vi "IMAQ FPGA Camera Link Pixel Bus to Vision Pixel Bus U16x1.vi"(5 "Reset Overflow":bool, 6 "Ready for Output":bool=TRUE, 7 "Overflow In":bool, 8 "Input Valid":bool=TRUE, 9 "Frame Valid In":bool, 10 "Line Valid In":bool, 11 "Pixel In":u16) -> (0 "Output Valid":bool, 2 "Acquisition Overflow":bool, 3 "Vision Pixel Bus Out":T1)   [LabVIEW 2017]
doc: "The Pixel Bus to Vision Pixel Bus takes the <B>Pixel In</B> and the timing signals (Line Valid, Frame Valid, and Input Valid) and converts them to the data structure used by Vision FPGA functions where the Line Valid and Frame Valid are part of the <B>Vision Pixel Bus Out</B> data structure.\n\nIf Ready For Output is ever False (i.e. downstream VIs are not ready for new pixel data), and this VI is about to output a valid Vision Pixel Bus, the Acquisition Overflow will assert and stay high to indicate pixel data was lost. The CameraLink pixel bus can not be slowed down, so the downstream processing VIs and transfer VIs need to ensure they can handle the CameraLink throughput to avoid missing pixels.\n\nThis VI requires a cycle to add End of Line and another cycle to add End of Image at the end of every image. This means there needs to be at least two blanking cycles between frames.s"
uses:
  <vilib>/visionFPGA/Controls/IMAQ FPGA Pixel Bus u16x1.ctl
  <vilib>/visionFPGA/Basics/Camera Link Acquisition/Controls/IMAQ FPGA Camera Link Pixel Bus to Vision Bus State.ctl
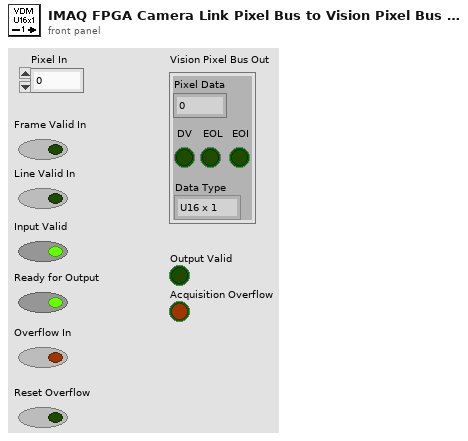
[diagram p1: front panel]
types:
  T1 = typedef "IMAQ FPGA Pixel Bus u16x1.ctl" = cluster{"Pixel Data":u16, "DV":bool, "EOL":bool, "EOI":bool, "Data Type":enum16{"U16 x 1"}}
  T2 = typedef "IMAQ FPGA Camera Link Pixel Bus to Vision Bus State.ctl" = enum16{"WaitForFirstPixel", "WaitForEndOfLine", "WaitForStartofNextLineOrEndOfImage", "HandleEndOfImage"}
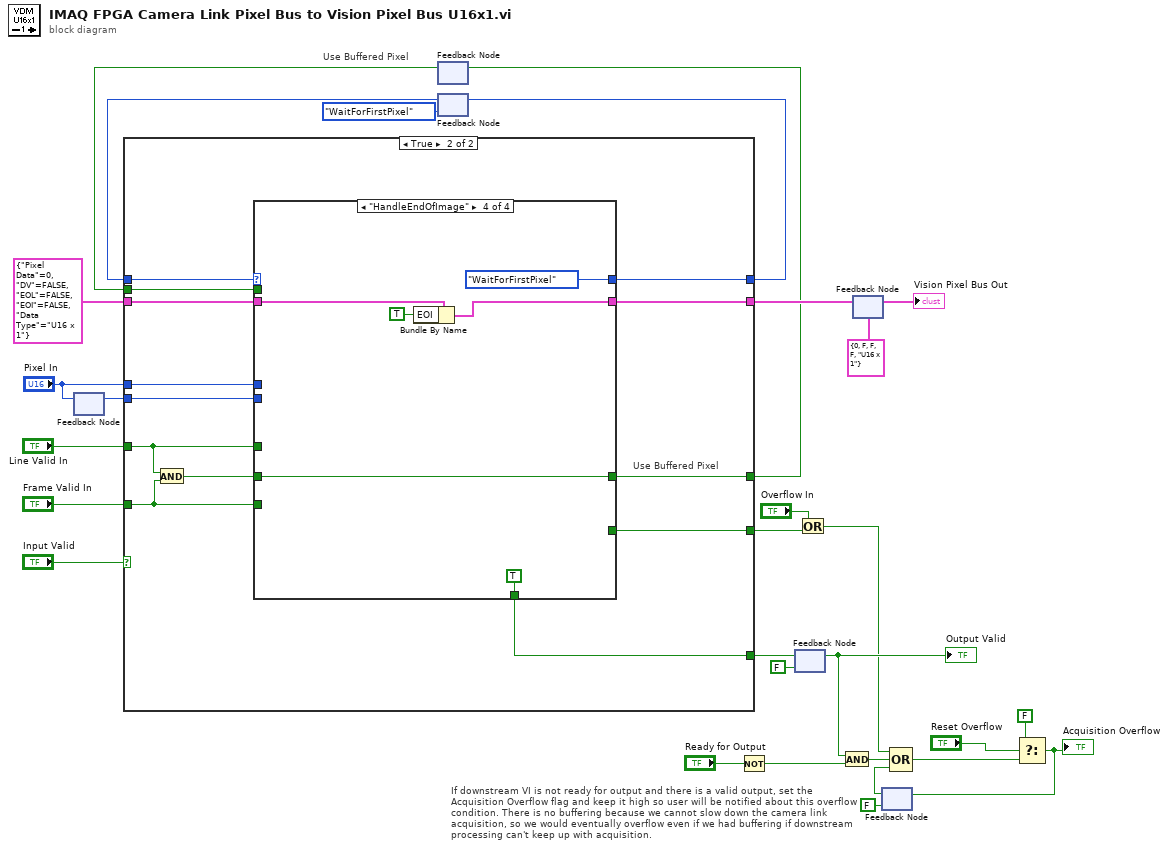
[diagram p0: block diagram]
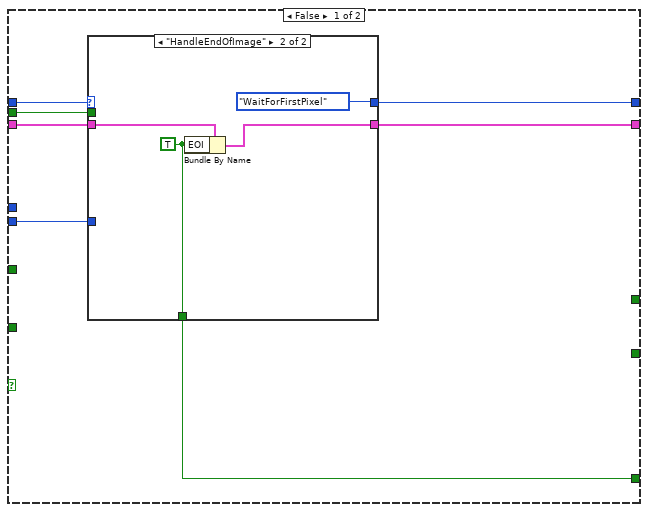
[diagram p2: hidden frame]
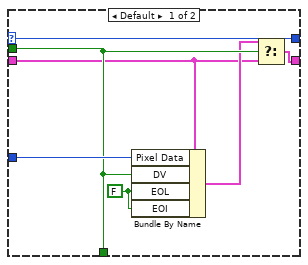
[diagram p3: hidden frame]
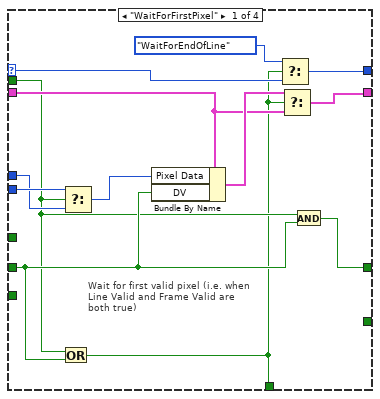
[diagram p4: hidden frame]
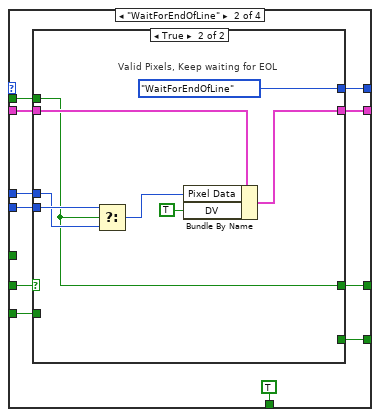
[diagram p5: hidden frame]
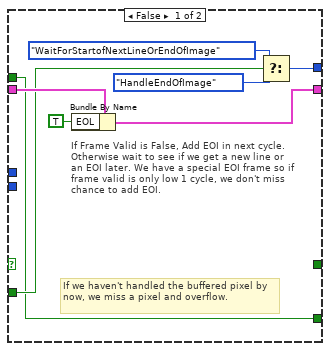
[diagram p6: hidden frame]
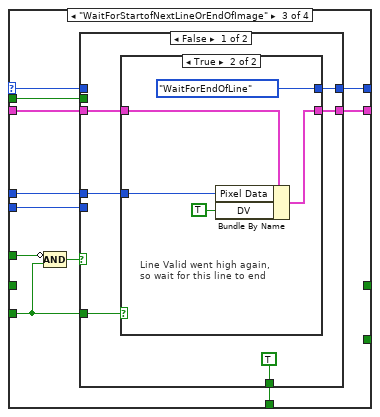
[diagram p7: hidden frame]
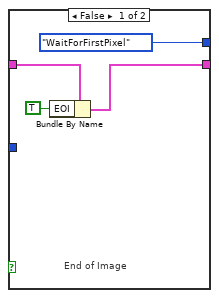
[diagram p8: hidden frame]
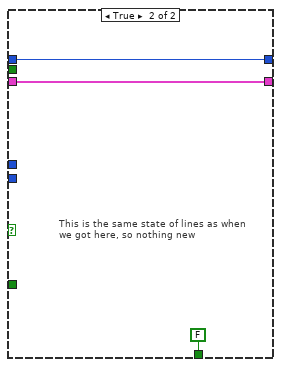
[diagram p9: hidden frame]
diagram:
  # "Use Buffered Pixel"
  # "If downstream VI is not ready for output and there is a valid output, set the Acquisition Overflow flag and keep it high so user will be notified about this overflow condition. There is no buffering because we cannot slow down the camera link acquisition, so we would eventually overflow even if we had buffering if downstream processing can't keep up with acquisition."
  n1 = feedback #1() -> (w7:u16)  [unwired: 1 in]
  n2 = feedback-in #1("Pixel In") -> ()
  n3 = feedback #2() -> (w8:bool)  [unwired: 1 in]
  n4 = feedback #3(IMAQ_FPGA_Camera_Link_Pixel_Bus_to_Vision_Bus_State."WaitForFirstPixel") -> (w11:T2)
  n5 = case shown="True" "Input Valid" {
    tunnel: [w32 w54] -> w25
    tunnel: "Line Valid In" -> [_ w56]
    tunnel: "Frame Valid In" -> [_ w55]
    tunnel: [w34 w59] -> w24
    tunnel: T1 {"Pixel Data"=0, "DV"=FALSE, "EOL"=FALSE, "EOI"=FALSE, "Data Type"=enum."U16 x 1"} ("Vision Pixel Bus Out") -> [w35 w60]
    tunnel: "Pixel In" -> [_ w58]
    tunnel: [w33 w53] -> w12
    tunnel: w11 -> [w36 w52]
    tunnel: [_ w51] -> w10
    tunnel: w8 -> [w31 w50]
    tunnel: w7 -> [w30 w49]
    tunnel: [_ w48] -> w5
    frame False {
      n6 = case shown="\"HandleEndOfImage\"" w36 {
        selector: w36 -> [w43 _]
        tunnel: w35 -> [w38 w47]
        tunnel: [w37 w46] -> w34
        tunnel: [w43 IMAQ_FPGA_Camera_Link_Pixel_Bus_to_Vision_Bus_State."WaitForFirstPixel"] -> w33
        tunnel: [w40 w44] -> w32
        tunnel: w31 -> [w40 _]
        tunnel: w30 -> [w42 _]
        frame Default {
          w41 = FALSE ("EOL")
          n7 = Bundle By Name(cluster=w38, "Pixel Data"=w42, "DV"=w40, "EOL"=w41, "EOI"=w41) -> (w39:T1)
          n8 = Select(t=w39, s=w40, f=w38) -> (s? t:f=w37:T1)
        }
        frame "HandleEndOfImage" {
          w44 = TRUE ("EOI")
          n9 = Bundle By Name(cluster=w47, "EOI"=w44) -> (w46:T1)
        }
      }
    }
    frame True {
      # "Use Buffered Pixel"
      n10 = And(x=w56, y=w55) -> (x .and. y?=w57:bool)
      n11 = case shown="\"HandleEndOfImage\"" w52 {
        selector: w52 -> [w72 _ w109 _]
        tunnel: [w73 w80 w108 IMAQ_FPGA_Camera_Link_Pixel_Bus_to_Vision_Bus_State."WaitForFirstPixel"] -> w53
        tunnel: w55 -> [_ w79 w104 _]
        tunnel: w56 -> [_ _ w106 _]
        tunnel: w60 -> [w68 w83 w111 w134]
        tunnel: [w71 w81 w110 w132] -> w59
        tunnel: w58 -> [w66 w82 w103 _]
        tunnel: w57 -> [w63 w84 _ w130]
        tunnel: [w61 TRUE w107 TRUE] -> w54
        tunnel: [w64 w75 _ w130] -> w51
        tunnel: w50 -> [w62 w77 w102 _]
        tunnel: w49 -> [w67 w76 w101 _]
        tunnel: [_ w74 _ _] -> w48
        frame "WaitForFirstPixel" {
          # "Wait for first valid pixel (i.e. when Line Valid and Frame Valid are both true)"
          n12 = Or(x=w62, y=w63) -> (x .or. y?=w61:bool)
          n13 = Select(t=w67, s=w62, f=w66) -> (s? t:f=w65:u16)
          n14 = Bundle By Name(cluster=w68, "Pixel Data"=w65, "DV"=w63) -> (w69:T1)
          n15 = Select(t=IMAQ_FPGA_Camera_Link_Pixel_Bus_to_Vision_Bus_State."WaitForEndOfLine", s=w61, f=w72) -> (s? t:f=w73:T2)
          n16 = Select(t=w69, s=w61, f=w68) -> (s? t:f=w71:T1)
          n17 = And(x=w62, y=w63) -> (x .and. y?=w64:bool)
        }
        frame "WaitForEndOfLine" {
          n18 = case shown="True" w84 {
            tunnel: w83 -> [w92 w100]
            tunnel: w82 -> [_ w95]
            tunnel: [w91 w99] -> w81
            tunnel: [w86 IMAQ_FPGA_Camera_Link_Pixel_Bus_to_Vision_Bus_State."WaitForEndOfLine"] -> w80
            tunnel: w79 -> [w89 _]
            tunnel: w77 -> [w85 w93]
            tunnel: w76 -> [_ w96]
            tunnel: [_ w93] -> w75
            tunnel: [w85 _] -> w74
            frame False {
              # "If we haven't handled the buffered pixel by now, we miss a pixel and overflow."
              # "If Frame Valid is False, Add EOI in next cycle. Otherwise wait to see if we get a new line or an EOI later. We have a special EOI frame so if frame valid is only low 1 cycle, we don't miss chance to add EOI."
              n19 = Bundle By Name(cluster=w92, "EOL"=TRUE) -> (w91:T1)
              n20 = Select(t=IMAQ_FPGA_Camera_Link_Pixel_Bus_to_Vision_Bus_State."WaitForStartofNextLineOrEndOfImage", s=w89, f=IMAQ_FPGA_Camera_Link_Pixel_Bus_to_Vision_Bus_State."HandleEndOfImage") -> (s? t:f=w86:T2)
            }
            frame True {
              # "Valid Pixels, Keep waiting for EOL"
              n21 = Select(t=w96, s=w93, f=w95) -> (s? t:f=w94:u16)
              n22 = Bundle By Name(cluster=w100, "Pixel Data"=w94, "DV"=TRUE) -> (w99:T1)
            }
          }
        }
        frame "WaitForStartofNextLineOrEndOfImage" {
          n23 = Compound Arithmetic op=AND(invert w106, w104) -> (w105:bool)
          n24 = case shown="False" w105 {
            tunnel: w111 -> [w116 w128]
            tunnel: [w115 w128] -> w110
            tunnel: w109 -> [_ w129]
            tunnel: [w114 w129] -> w108
            tunnel: [TRUE FALSE] -> w107
            tunnel: w104 -> [w113 _]
            tunnel: w103 -> [w112 _]
            tunnel: w102 -> [_ _]
            tunnel: w101 -> [_ _]
            frame False {
              n25 = case shown="True" w113 {
                tunnel: w116 -> [w121 w125]
                tunnel: [w119 w124] -> w115
                tunnel: [IMAQ_FPGA_Camera_Link_Pixel_Bus_to_Vision_Bus_State."WaitForFirstPixel" IMAQ_FPGA_Camera_Link_Pixel_Bus_to_Vision_Bus_State."WaitForEndOfLine"] -> w114
                tunnel: w112 -> [_ w123]
                frame False {
                  # "End of Image"
                  n26 = Bundle By Name(cluster=w121, "EOI"=TRUE) -> (w119:T1)
                }
                frame True {
                  # "Line Valid went high again, so wait for this line to end"
                  n27 = Bundle By Name(cluster=w125, "Pixel Data"=w123, "DV"=TRUE) -> (w124:T1)
                }
              }
            }
            frame True {
              # "This is the same state of lines as when we got here, so nothing new"
            }
          }
        }
        frame "HandleEndOfImage" {
          n28 = Bundle By Name(cluster=w134, "EOI"=TRUE) -> (w132:T1)
        }
      }
    }
  }
  n29 = feedback-in #2(w10) -> ()
  n30 = feedback-in #3(w12) -> ()
  n31 = Not(x="Ready for Output") -> (.not. x?=w22:bool)
  n32 = feedback #4(FALSE) -> (w21:bool)
  "Output Valid" <- w21
  n33 = feedback-in #4(w25) -> ()
  n34 = Or(x="Overflow In", y=w5) -> (x .or. y?=w4:bool)
  n35 = And(x=w21, y=w22) -> (x .and. y?=w20:bool)
  n36 = feedback #5(T1 {"Pixel Data"=0, "DV"=FALSE, "EOL"=FALSE, "EOI"=FALSE, "Data Type"=enum."U16 x 1"} ("Vision Pixel Bus Out")) -> (→"Vision Pixel Bus Out":T1)
  n37 = feedback-in #5(w24) -> ()
  n38 = feedback #6(FALSE) -> (w19:bool)
  n39 = Compound Arithmetic op=OR(w4, w20, w19) -> (w16:bool)
  n40 = Select(t=FALSE, s="Reset Overflow", f=w16) -> (s? t:f=w15:bool)
  "Acquisition Overflow" <- w15
  n41 = feedback-in #6(w15) -> ()
